vi "Servo Angle Set.vi"(5 "Servo Angle Set":dbl, 11 "error in (no error)":errorcluster) -> (15 "error out (no error)":errorcluster)   [LabVIEW 2013]
uses:
  Camera/Camera Global Data.vi
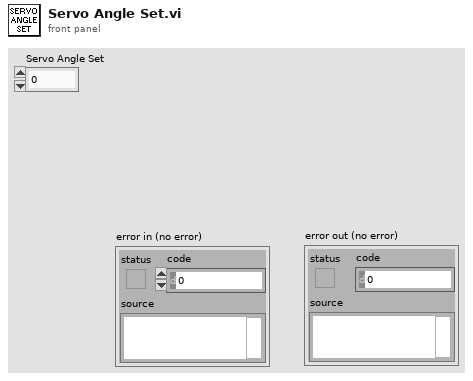
[diagram p1: front panel]
types:
  T1 = cluster{"Servo Angle Get":dbl, "Servo Angle Set":dbl}
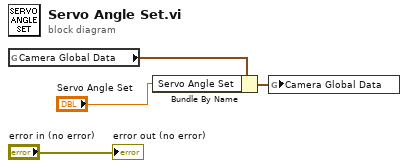
[diagram p0: block diagram]
diagram:
  n1 = global read "Camera Global Data.vi" "Camera Global Data"() -> (w4:T1)
  n2 = Bundle By Name(cluster=w4, "Servo Angle Set"="Servo Angle Set") -> (w3:T1)
  n3 = global write "Camera Global Data.vi" "Camera Global Data"(w3) -> ()
  "error out (no error)" <- "error in (no error)"
